vi "Write Libary Refnum.vi"(8 "error in (no error)":errorcluster, 10 "Libary Refnum":refnum<vi>, 11 "TestRunner in":refnum<class "TestRunner.lvclass">) -> (0 "error out":errorcluster, 3 "TestRunner out":refnum<class "TestRunner.lvclass">)   [LabVIEW 2019, in "TestRunner.lvlib" / "TestRunner.lvclass"]
uses:
  TestRunner.lvclass
  TestRunner.lvclass/TestRunner.ctl
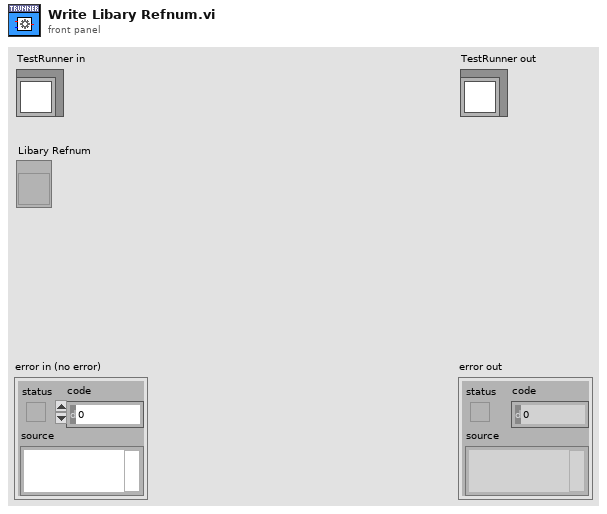
[diagram p1: front panel]
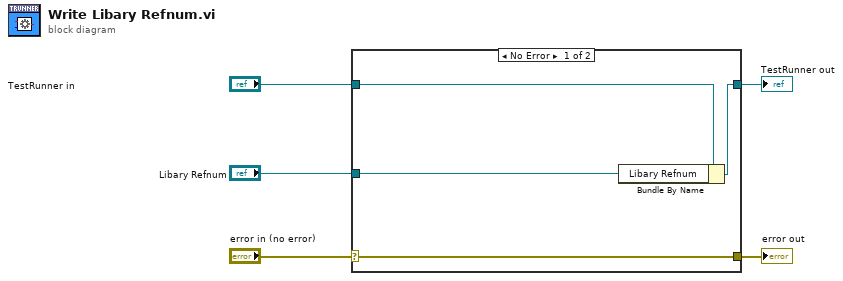
[diagram p0: block diagram]
diagram:
  n1 = case shown="No Error" "error in (no error)" {
    selector: "error in (no error)" -> [w9 w10]
    tunnel: [w9 w10] -> w4
    tunnel: [w7 w11] -> w2
    tunnel: "TestRunner in" -> [w8 w11]
    tunnel: "Libary Refnum" -> [w6 _]
    frame No Error {
      n2 = Bundle By Name(cluster=w8, "Libary Refnum"=w6) -> (w7:refnum<class "TestRunner.lvclass">)
    }
    frame Error {
    }
  }
  "error out" <- w4
  "TestRunner out" <- w2
